vi "Get Emb Model Name.vi"(11 "Embedding Model Name in":string caption="Embedding Model URL in") -> (3 "Embedding Model Name out":string)   [LabVIEW 2023, in "LabVIEW RAG.lvlib"]
uses:
  LabVIEW RAG.lvlib
  AI RAG Globals.vi
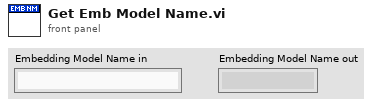
[diagram p1: front panel]
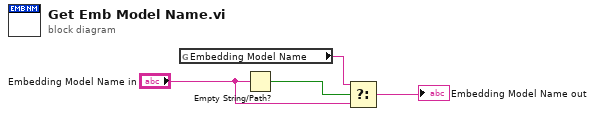
[diagram p0: block diagram]
diagram:
  n1 = global read "AI RAG Globals.vi" "Embedding Model Name"() -> (w4:string)
  n2 = Empty String/Path?(string/path="Embedding Model Name in") -> (empty?=w3:bool)
  n3 = Select(t=w4, s=w3, f="Embedding Model Name in") -> (s? t:f=→"Embedding Model Name out":string)
